vi "Length_10.vi"() -> ()   [LabVIEW 2020]
uses:
  Support/Controls/Cmd_Mouse Popup.ctl
  Support/Controls/Clst_Initialize Input.ctl
  Support/Controls/Clst_Result inspec.ctl
  Support/Controls/Cmd_Var Data IO.ctl
  Variables/Global_Cal Info.vi
panel:
  in  "주파수단위":string(combo)="kHz"
  in  "주파수":string
  in  "입력단위":string(combo)="DC"
  in  "Measured ADJ":string[][](table) caption="조정후"
  out "STD set":string[][](table) caption="○ 기준기 조합 (값)"
  in  "입력전압":dbl=10.0
  in  "정격출력":dbl=10.0
  in  "최소출력":dbl
  in  "출력단위":string(combo)="V"
  out "최소범위":string
  out "Resolution":string[][](table) caption="Spec"
  in  "Spec 변경":bool
  in  "Random":bool
  out "Spec":string[][](table)
  out "제목":string
  out "에러 출력":errorcluster
  out "Condition":string[][](table)
  out "최소눈금":string
  out "단위":string
  out "최대범위":string
  in  "Measured":string[][](table) caption="조정전"
  out "Load?":bool
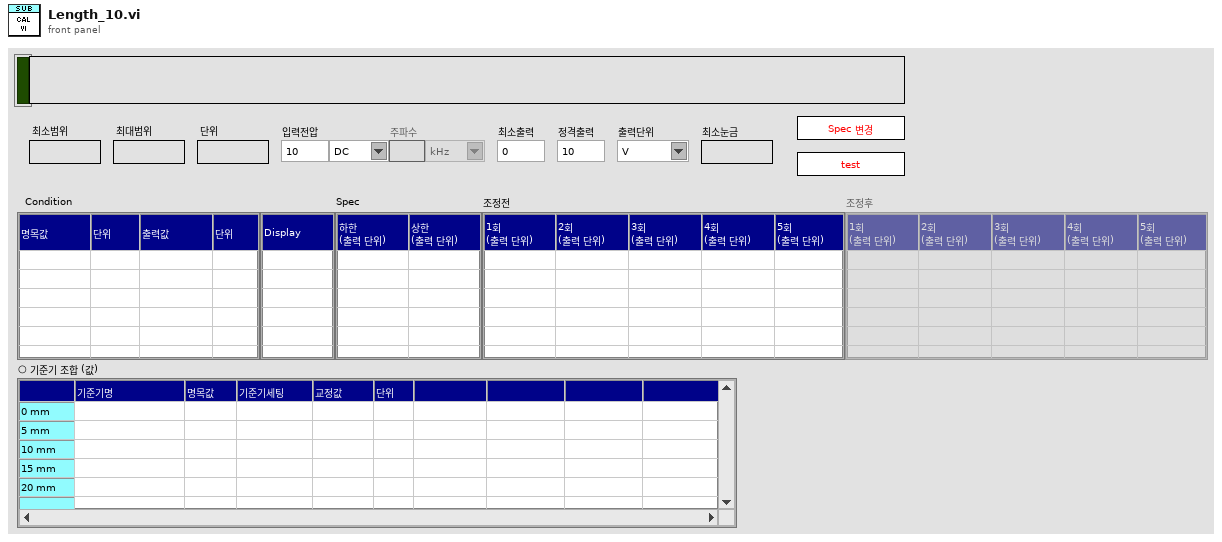
[diagram p1: front panel]
types:
  T1 = typedef "Cmd_Mouse Popup.ctl" = enum16{"활성화", "메뉴선택"}
  T2 = cluster{"Shift":bool, "Ctrl":bool, "Alt":bool, "Cmd":bool, "Opt":bool}
  T3 = typedef "Clst_Initialize Input.ctl" = cluster{"Initialize 1":cluster{"Condition":refnum<vi>[], "Spec":refnum<vi>[], "Measured":refnum<vi>[], "Resolution":refnum<vi>[], "Func_ext":string, "제목":refnum<vi>, "Measured_ADJ":refnum<vi>[]}, "Initialize 2":cluster{"문자열":refnum<vi>[], "콤보박스":refnum<vi>[], "링":refnum<vi>[], "열거형":refnum<vi>[], "테이블":refnum<vi>[], "여러열":refnum<vi>[], "디지털(DBL)":refnum<vi>[], "3D string":refnum<vi>[], "ctrl":refnum<vi>[], "boolean":refnum<vi>[]}}
  T4 = typedef "Clst_Result inspec.ctl" = cluster{"분해능":string, "문자열 1":string, "문자열 2":string, "숫자형 1":i32, "숫자형 2":i32, "숫자형 3":dbl, "문자배열 1D":string[], "문자배열 2D":string[][], "문자배열 3D":string[][][], "문자배열 4D":string[][][][], "불리언 1D":bool[]}
  T5 = typedef "Cmd_Var Data IO.ctl" = enum16{"Condition", "Condition Default", "Condition_Temp", "Resolution", "Resolution Default", "Resolution Old", "Spec", "Spec Default", "Spec Old", "Spec Temp", "Result", "Result2", "Result3", "Result_Temp", "Result_ADJ", "Result_ADJ2", "STD1", "STD2", "STD3", "STD4", "STD5", "STD Temp", "CMC", "CMC Default"}
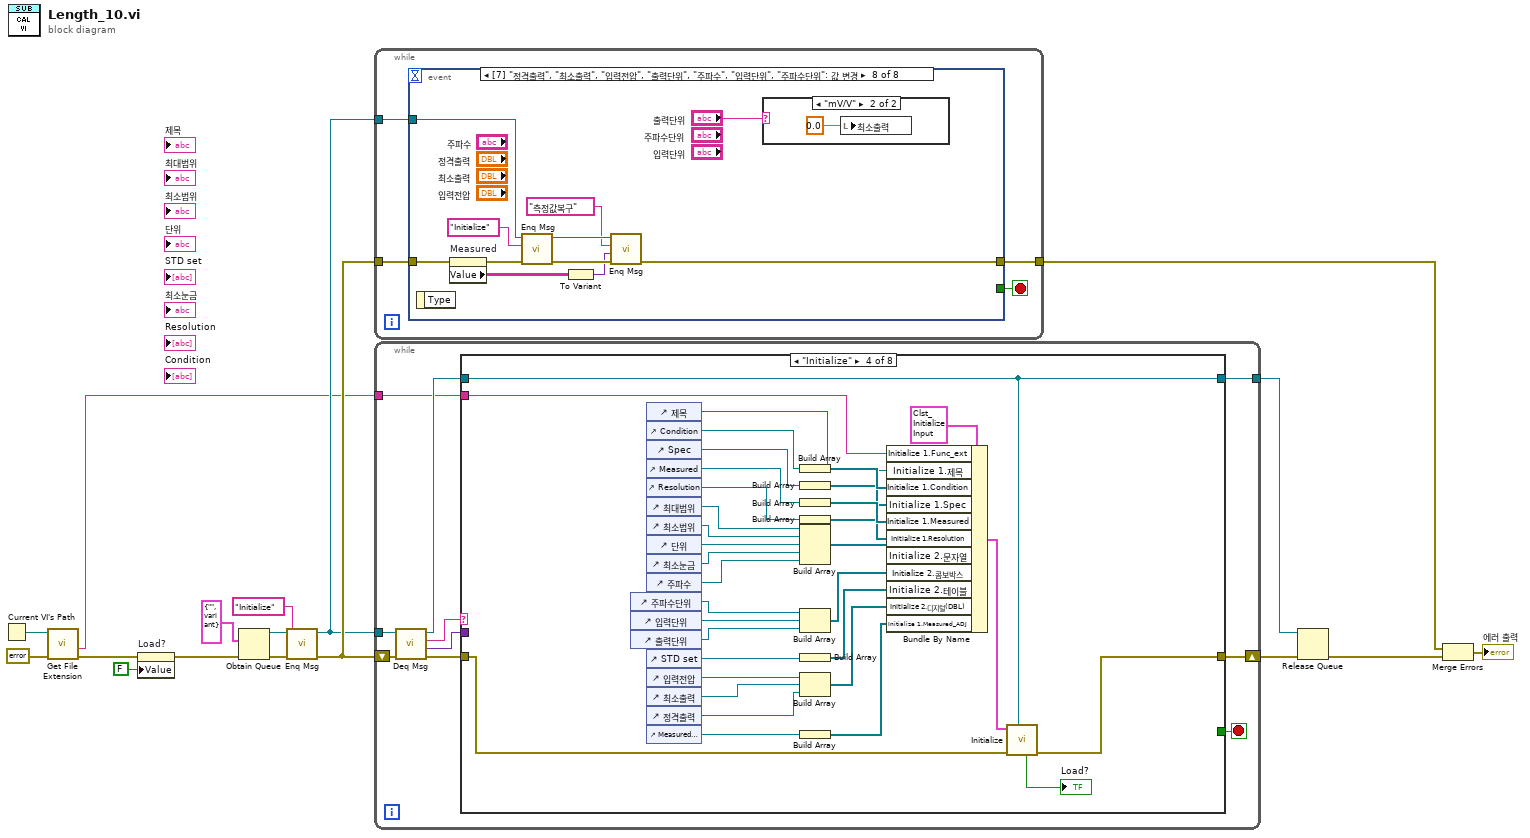
[diagram p0: block diagram]
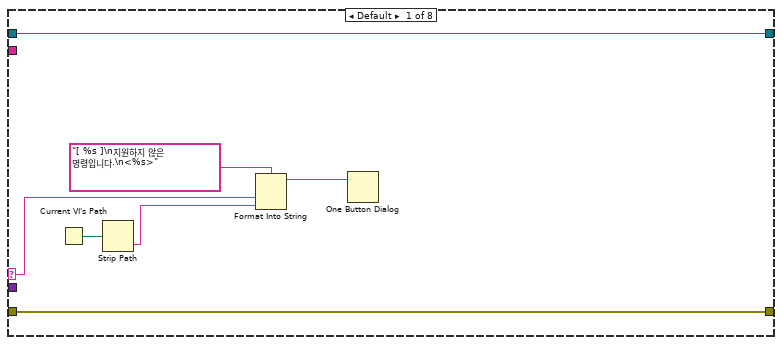
[diagram p2: hidden frame]
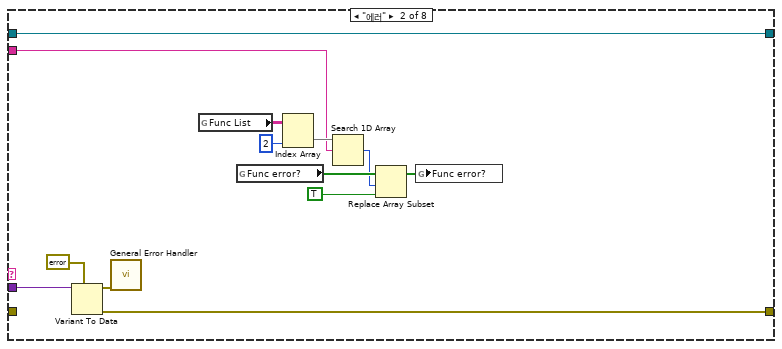
[diagram p3: hidden frame]
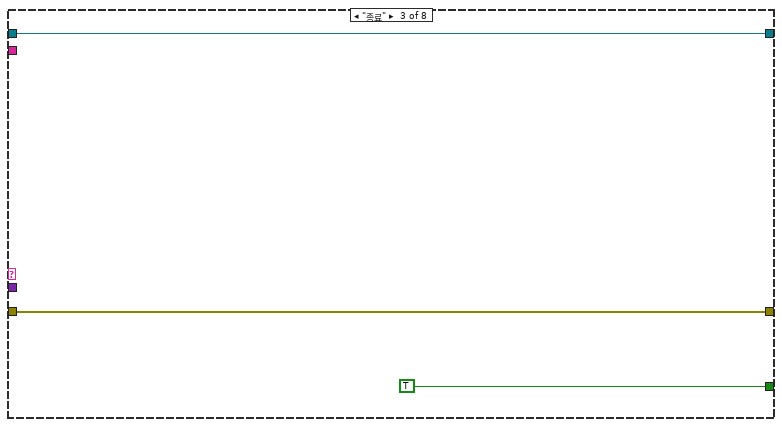
[diagram p4: hidden frame]
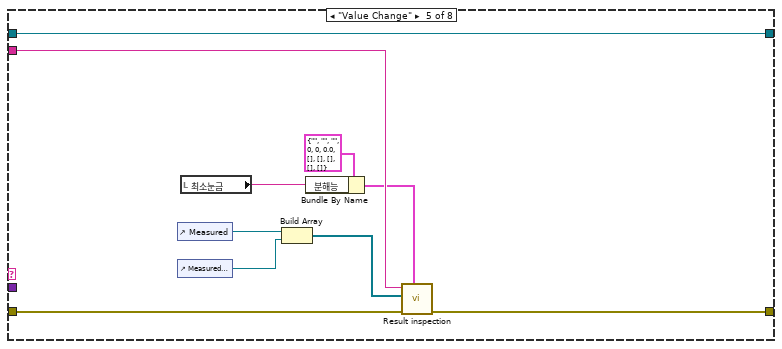
[diagram p5: hidden frame]
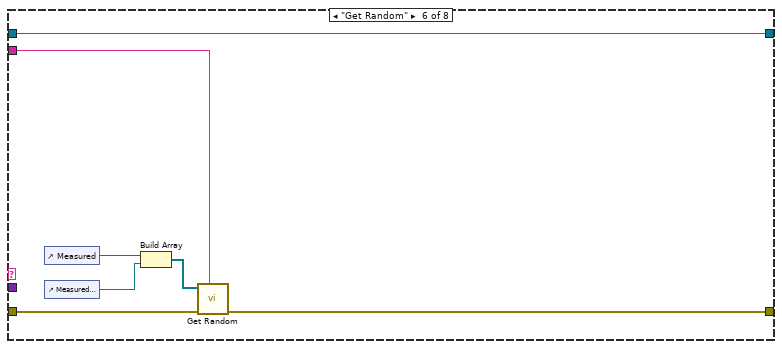
[diagram p6: hidden frame]
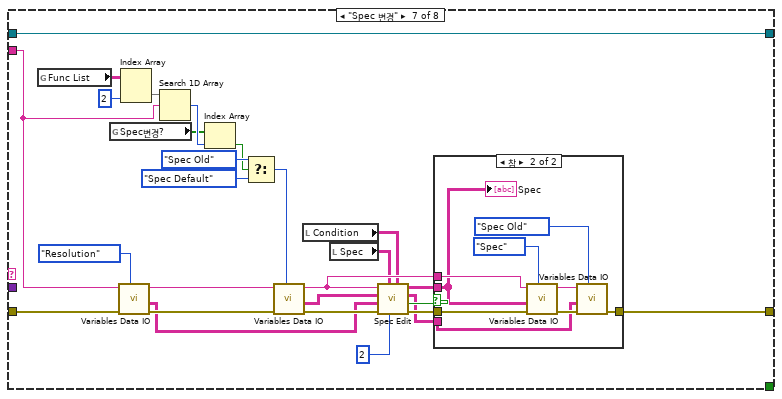
[diagram p7: hidden frame]
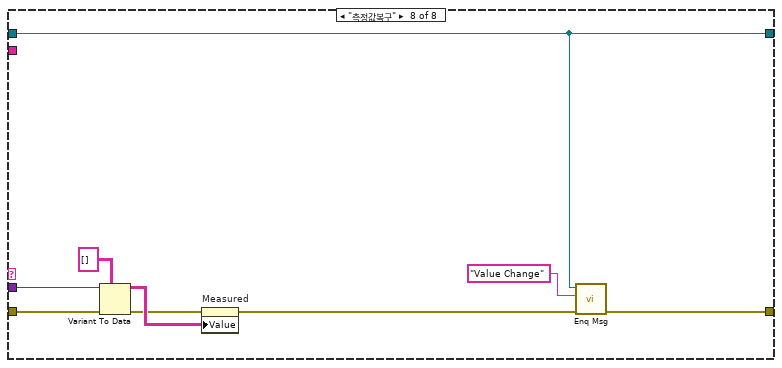
[diagram p9: hidden frame]
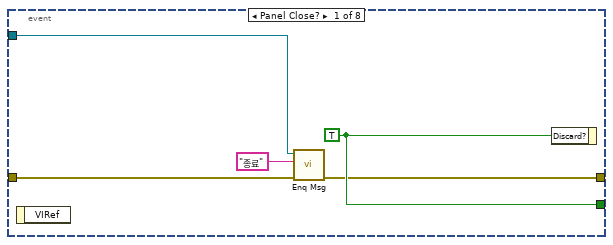
[diagram p10: hidden frame]
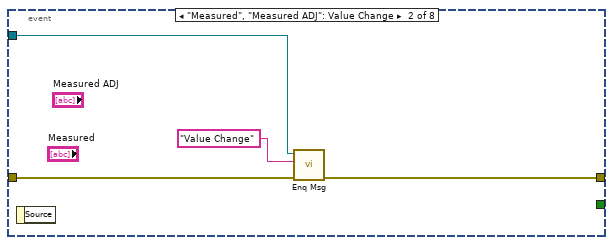
[diagram p11: hidden frame]
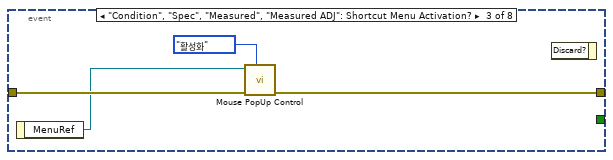
[diagram p12: hidden frame]
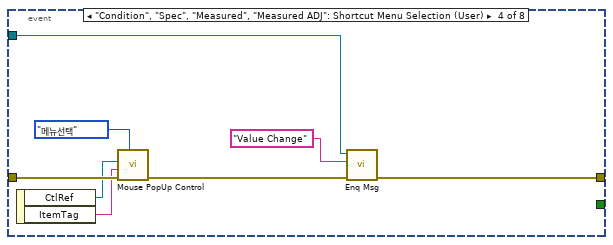
[diagram p13: hidden frame]
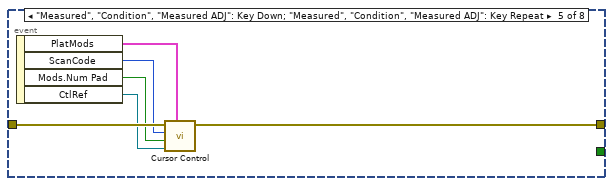
[diagram p14: hidden frame]
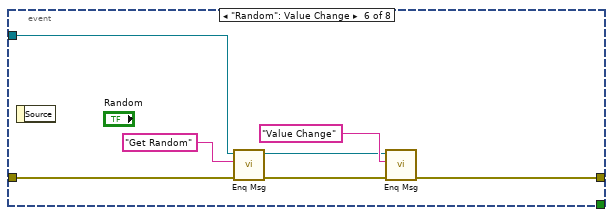
[diagram p15: hidden frame]
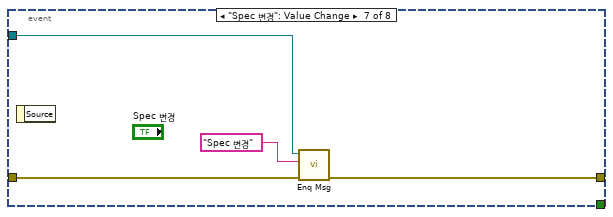
[diagram p16: hidden frame]
diagram:
  n1 = Current VI's Path() -> (path=w7:path)
  n2 = call <vilib>:"Get File Extension.vi"("error in (no error)"=errorcluster {"status"=FALSE, "code"=0, "source"=""} ("에러 상수"), "file"=w7) -> ("error out"=w3:errorcluster, "filename without extension"=w6:string)  [unwired: 5 in, 3 out]
  n3 = property on="Load?" class="Bool (엄격한)"(error in=w3, "Value"=FALSE ("Load?")) -> (error out=w2:errorcluster)  [unwired: 1 in, 1 out]
  n4 = Obtain Queue(element data type=cluster{"메세지":string, "값":variant} {"메세지"="", "값"=variant} ("Message Cluster"), error in (no error)=w2) -> (queue out=w15:refnum<queue>, error out=w5:errorcluster)  [unwired: 3 in, 1 out]
  n5 = call "Enq Msg.vi"("에러 입력(에러 없음)"=w5, "메세지"="Initialize", "큐 입력"=w15) -> ("에러 출력"=w16:errorcluster, "큐 출력"=w13:refnum<queue>)  [unwired: 7 in]
  n6 = while {
    tunnel: w16 -> [w19]
    tunnel: w13 -> [w20]
    tunnel: [w18] -> w10
    stop <- w21 stop-if-true
    n7 = event shown="[7] \"정격출력\", \"최소출력\", \"입력전압\", \"출력단위\", \"주파수\", \"입력단위\", \"주파수단위\": 값 변경" {
      selector: _ -> [_ _ _ _ _ _ _ _]
      dyn-events: _ -> [_ _ _ _ _ _ _ _]
      timeout: _ -> [_ _ _ _ _ _ _ _]
      tunnel: [w26 _ _ _ _ _ _ _] -> w21
      tunnel: w20 -> [w24 w29 _ w37 _ w50 w56 w69]
      tunnel: w19 -> [w25 w30 w33 w41 w48 w51 w58 w67]
      tunnel: [w22 w28 w32 w36 w47 w49 w57 w60] -> w18
      event Panel Close? {
        w26 = TRUE ("버림?")
        n8 = event-data() -> ()  [unwired: 1 in, 1 out]
        n9 = call "Enq Msg.vi"("에러 입력(에러 없음)"=w25, "메세지"="종료", "큐 입력"=w24) -> ("에러 출력"=w22:errorcluster)  [unwired: 7 in, 1 out]
        n10 = event-data("Discard?"=w26) -> ()  [unwired: 1 in, 1 out]
      }
      event "Measured", "Measured ADJ": Value Change {
        n11 = event-data() -> ()  [unwired: 1 in, 1 out]
        n12 = call "Enq Msg.vi"("에러 입력(에러 없음)"=w30, "메세지"="Value Change", "큐 입력"=w29) -> ("에러 출력"=w28:errorcluster)  [unwired: 7 in, 1 out]
      }
      event "Condition", "Spec", "Measured", "Measured ADJ": Shortcut Menu Activation? {
        n13 = event-data() -> ("MenuRef"=w31:refnum<k9>)  [unwired: 1 in]
        n14 = call "Mouse PopUp Control.vi"("type"=Cmd_Mouse_Popup."활성화", "error in"=w33, "메뉴 참조"=w31) -> ("error out"=w32:errorcluster)  [unwired: 8 in]
        n15 = event-data() -> ()  [unwired: 2 in, 1 out]
      }
      event "Condition", "Spec", "Measured", "Measured ADJ": Shortcut Menu Selection (User) {
        n16 = event-data() -> ("CtlRef"=w39:refnum<vi>, "ItemTag"=w40:string)  [unwired: 1 in]
        n17 = call "Mouse PopUp Control.vi"("type"=Cmd_Mouse_Popup."메뉴선택", "error in"=w41, "아이템 태그"=w40, "Tbl 참조 번호"=w39) -> ("error out"=w38:errorcluster)  [unwired: 7 in]
        n18 = call "Enq Msg.vi"("에러 입력(에러 없음)"=w38, "메세지"="Value Change", "큐 입력"=w37) -> ("에러 출력"=w36:errorcluster)  [unwired: 7 in, 1 out]
      }
      event "Measured", "Condition", "Measured ADJ": Key Down; "Measured", "Condition", "Measured ADJ": Key Repeat {
        n19 = event-data() -> ("PlatMods"=w43:T2, "ScanCode"=w46:i16, "Mods.Num Pad"=w45:bool, "CtlRef"=w44:refnum<vi>)  [unwired: 1 in]
        n20 = call "Cursor Control.vi"("플랫폼 조합키"=w43, "참조"=w44, "Num Pad"=w45, "ScanCode"=w46, "error in"=w48) -> ("error out"=w47:errorcluster)  [unwired: 5 in, 1 out]
      }
      event "Random": Value Change {
        n21 = event-data() -> ()  [unwired: 1 in, 1 out]
        n22 = call "Enq Msg.vi"("에러 입력(에러 없음)"=w51, "메세지"="Get Random", "큐 입력"=w50) -> ("에러 출력"=w53:errorcluster, "큐 출력"=w54:refnum<queue>)  [unwired: 7 in]
        n23 = call "Enq Msg.vi"("에러 입력(에러 없음)"=w53, "메세지"="Value Change", "큐 입력"=w54) -> ("에러 출력"=w49:errorcluster)  [unwired: 7 in, 1 out]
      }
      event "Spec 변경": Value Change {
        n24 = event-data() -> ()  [unwired: 1 in, 1 out]
        n25 = call "Enq Msg.vi"("에러 입력(에러 없음)"=w58, "메세지"="Spec 변경", "큐 입력"=w56) -> ("에러 출력"=w57:errorcluster)  [unwired: 7 in, 1 out]
      }
      event "정격출력", "최소출력", "입력전압", "출력단위", "주파수", "입력단위", "주파수단위": Value Change {
        n26 = event-data() -> ()  [unwired: 1 in, 1 out]
        n27 = property on="Measured" class="Tbl (엄격한)"(error in=w67) -> (error out=w66:errorcluster, "Value"=w63:string[][])  [unwired: 1 in, 1 out]
        n28 = call "Enq Msg.vi"("에러 입력(에러 없음)"=w66, "메세지"="Initialize", "큐 입력"=w69) -> ("에러 출력"=w65:errorcluster, "큐 출력"=w68:refnum<queue>)  [unwired: 7 in]
        n29 = To Variant(anything=w63) -> (Variant=w62:variant)
        n30 = call "Enq Msg.vi"("에러 입력(에러 없음)"=w65, "값"=w62, "메세지"="측정값복구", "큐 입력"=w68) -> ("에러 출력"=w60:errorcluster)  [unwired: 6 in, 1 out]
        n31 = case shown="\"mV/V\"" "출력단위" {
          frame Default {
          }
          frame "mV/V" {
            n32 = local write "최소출력"(0.0 ("최소출력")) -> ()
          }
        }
      }
    }
  }
  n33 = while {
    shift-right: [w81] -> w12
    shift-left: w16 -> [w80]
    tunnel: w13 -> [w78]
    tunnel: [w73] -> w11
    tunnel: w6 -> [w72]
    stop <- w74 stop-if-true
    n34 = call "Deq Msg.vi"("에러 입력(에러 없음)"=w80, "큐 입력"=w78) -> ("에러 출력"=w79:errorcluster, "값"=w75:variant, "메세지"=w77:string, "큐 출력"=w76:refnum<queue>)  [unwired: 6 in]
    n35 = case shown="\"Initialize\"" w77 {
      selector: w77 -> [w84 _ _ _ _ _ _ _]
      tunnel: w79 -> [w88 _ w104 w113 w145 w153 w176 w199]
      tunnel: [w88 w98 w104 w112 w147 w150 w180 w194] -> w81
      tunnel: w76 -> [w87 w97 w102 w125 w148 w155 w182 w193]
      tunnel: w75 -> [_ w99 _ _ _ _ _ w198]
      tunnel: [_ _ TRUE ("버림?") _ _ _ _ _] -> w74
      tunnel: [w87 w97 w102 w125 w148 w155 w182 w193] -> w73
      tunnel: w72 -> [_ w89 _ w121 w146 w151 w157 _]
      frame Default {
        n36 = Current VI's Path() -> (path=w83:path)
        n37 = Strip Path(path=w83) -> (name=w82:string)  [unwired: 1 out]
        n38 = Format Into String(format string="[ %s ]\n지원하지 않은 명령입니다.\n<%s>" ("메시지"), w84, w82) -> (resulting string=w85:string)  [unwired: 2 in, 1 out]
        n39 = One Button Dialog(message=w85) -> ()  [unwired: 1 in, 1 out]
      }
      frame "에러" {
        n40 = Variant To Data(type=errorcluster {"status"=FALSE, "code"=0, "source"=""} ("에러 출력"), Variant=w99) -> (data=w101:errorcluster, error out=w98:errorcluster)  [unwired: 1 in]
        n41 = call <vilib>:"General Error Handler.vi"("error in (no error)"=w101) -> ()  [unwired: 10 in, 5 out]
        n42 = global read "Global_Cal Info.vi" "Func List"() -> (w95:string[][])
        n43 = global read "Global_Cal Info.vi" "Func error?"() -> (w92:bool[])
        n44 = Index Array(array=w95, index (col)=2 ("비활성화된 인덱스 (열)")) -> (element=w94:string[])  [unwired: 1 in]
        n45 = Search 1D Array(1D array=w94, element=w89) -> (index of element=w91:i32)  [unwired: 1 in]
        n46 = Replace Array Subset(array=w92, new element=TRUE ("새 원소/부분배열"), index=w91) -> (w90:bool[])
        n47 = global write "Global_Cal Info.vi" "Func error?"(w90) -> ()
      }
      frame "종료" {
      }
      frame "Initialize" {
        n48 = control-ref of="주파수단위"() -> (w106:refnum<vi>)
        n49 = control-ref of="입력단위"() -> (w105:refnum<vi>)
        n50 = control-ref of="출력단위"() -> (w107:refnum<vi>)
        n51 = control-ref of="제목"() -> (w130:refnum<vi>)
        n52 = control-ref of="Condition"() -> (w136:refnum<vi>)
        n53 = control-ref of="Spec"() -> (w127:refnum<vi>)
        n54 = control-ref of="Measured"() -> (w133:refnum<vi>)
        n55 = control-ref of="Resolution"() -> (w124:refnum<vi>)
        n56 = control-ref of="최대범위"() -> (w129:refnum<vi>)
        n57 = control-ref of="최소범위"() -> (w120:refnum<vi>)
        n58 = control-ref of="단위"() -> (w128:refnum<vi>)
        n59 = control-ref of="최소눈금"() -> (w119:refnum<vi>)
        n60 = control-ref of="주파수"() -> (w108:refnum<vi>)
        n61 = control-ref of="STD set"() -> (w114:refnum<vi>)
        n62 = control-ref of="입력전압"() -> (w118:refnum<vi>)
        n63 = control-ref of="최소출력"() -> (w117:refnum<vi>)
        n64 = control-ref of="정격출력"() -> (w116:refnum<vi>)
        n65 = control-ref of="Measured ADJ"() -> (w111:refnum<vi>)
        n66 = Build Array(w136) -> (w135:refnum<vi>[])
        n67 = Build Array(w127) -> (w126:refnum<vi>[])
        n68 = Build Array(w133) -> (w134:refnum<vi>[])
        n69 = Build Array(w124) -> (w123:refnum<vi>[])
        n70 = Build Array(w129, w120, w128, w119, w108) -> (w132:refnum<vi>[])
        n71 = Build Array(w106, w105, w107) -> (w131:refnum<vi>[])
        n72 = Build Array(w114) -> (w122:refnum<vi>[])
        n73 = Build Array(w118, w117, w116) -> (w115:refnum<vi>[])
        n74 = Build Array(w111) -> (w110:refnum<vi>[])
        n75 = Bundle By Name(cluster=T3 {"Initialize 1"={"Condition"=[], "Spec"=[], "Measured"=[], "Resolution"=[], "Func_ext"="", "제목"=refnum, "Measured_ADJ"=[]}, "Initialize 2"={"문자열"=[], "콤보박스"=[], "링"=[], "열거형"=[], "테이블"=[], "여러열"=[], "디지털(DBL)"=[], "3D string"=[], "ctrl"=[], "boolean"=[]}} ("입력 클러스터"), "Initialize 1.Func_ext"=w121, "Initialize 1.제목"=w130, "Initialize 1.Condition"=w135, "Initialize 1.Spec"=w126, "Initialize 1.Measured"=w134, "Initialize 1.Resolution"=w123, "Initialize 2.문자열"=w132, "Initialize 2.콤보박스"=w131, "Initialize 2.테이블"=w122, "Initialize 2.디지털(DBL)"=w115, "Initialize 1.Measured_ADJ"=w110) -> (w137:T3)
        n76 = call "Initialize.vi"("큐 입력"=w125, "error in"=w113, "입력 클러스터"=w137) -> ("error out"=w112:errorcluster, "Load?"=→"Load?":bool)  [unwired: 5 in, 2 out]
      }
      frame "Value Change" {
        n77 = control-ref of="Measured"() -> (w144:refnum<vi>)
        n78 = control-ref of="Measured ADJ"() -> (w139:refnum<vi>)
        n79 = local read "최소눈금"() -> (w141:string)
        n80 = Build Array(w144, w139) -> (w143:refnum<vi>[])
        n81 = Bundle By Name(cluster=T4 {"분해능"="", "문자열 1"="", "문자열 2"="", "숫자형 1"=0, "숫자형 2"=0, "숫자형 3"=0.0, "문자배열 1D"=[], "문자배열 2D"=[], "문자배열 3D"=[], "문자배열 4D"=[], "불리언 1D"=[]} ("입력 클러스터"), "분해능"=w141) -> (w140:T4)
        n82 = call "Result inspection.vi"("입력 클러스터"=w140, "error in"=w145, "Ref. Data (Inspection)"=w143, "Func ext"=w146) -> ("error out"=w147:errorcluster)  [unwired: 4 in, 3 out]
      }
      frame "Get Random" {
        n83 = control-ref of="Measured"() -> (w152:refnum<vi>)
        n84 = control-ref of="Measured ADJ"() -> (w149:refnum<vi>)
        n85 = Build Array(w152, w149) -> (w154:refnum<vi>[])
        n86 = call "Get Random.vi"("Func_Ext"=w151, "에러 입력"=w153, "Meas"=w154) -> ("에러 출력"=w150:errorcluster)  [unwired: 7 in, 1 out]
      }
      frame "Spec 변경" {
        n87 = global read "Global_Cal Info.vi" "Func List"() -> (w162:string[][])
        n88 = global read "Global_Cal Info.vi" "Spec변경?"() -> (w158:bool[])
        n89 = call "Variables Data IO.vi"("Select"=Cmd_Var_Data_IO."Resolution", "error in"=w176, "Func_ext"=w157) -> ("error out"=w175:errorcluster, "Data Out"=w169:string[][], "Func_ext Out"=w174:string)  [unwired: 6 in]
        n90 = Index Array(array=w162, index (col)=2 ("비활성화된 인덱스 (열)")) -> (element=w160:string[])  [unwired: 1 in]
        n91 = Search 1D Array(1D array=w160, element=w157) -> (index of element=w159:i32)  [unwired: 1 in]
        n92 = Index Array(array=w158, index=w159) -> (element=w163:bool)
        n93 = Select(t=Cmd_Var_Data_IO."Spec Old" ("Select"), s=w163, f=Cmd_Var_Data_IO."Spec Default" ("Select")) -> (s? t:f=w156:T5)
        n94 = call "Variables Data IO.vi"("Select"=w156, "error in"=w175, "Func_ext"=w174) -> ("error out"=w177:errorcluster, "Data Out"=w168:string[][], "Func_ext Out"=w170:string)  [unwired: 6 in]
        n95 = local read "Condition"() -> (w166:string[][])
        n96 = local read "Spec"() -> (w167:string[][])
        n97 = call "Spec Edit.vi"("Condition"=w166, "열번호(기준값)"=2 ("기준열(0)"), "Spec Value"=w167, "에러 입력(에러 없음)"=w177, "Resolution"=w169, "Spec Default"=w168, "Func_ext"=w170) -> ("에러 출력"=w181:errorcluster, "변경?"=w178:bool, "Spec Default out"=w172:string[][], "Spec 출력"=w179:string[][])  [unwired: 1 in]
        n98 = case shown="참" w178 {
          tunnel: w181 -> [w183 w191]
          tunnel: [w183 w187] -> w180
          tunnel: w179 -> [_ w189]
          tunnel: w170 -> [_ w190]
          tunnel: w172 -> [_ w185]
          frame False {
          }
          frame True {
            n99 = call "Variables Data IO.vi"("Select"=Cmd_Var_Data_IO."Spec", "error in"=w191, "Data In"=w189, "Func_ext"=w190) -> ("error out"=w188:errorcluster, "Func_ext Out"=w186:string)  [unwired: 5 in, 1 out]
            n100 = call "Variables Data IO.vi"("Select"=Cmd_Var_Data_IO."Spec Old", "error in"=w188, "Data In"=w185, "Func_ext"=w186) -> ("error out"=w187:errorcluster)  [unwired: 5 in, 2 out]
            "Spec" <- w189
          }
        }
      }
      frame "측정값복구" {
        n101 = Variant To Data(error in=w199, type=string[][] [], Variant=w198) -> (data=w197:string[][], error out=w196:errorcluster)
        n102 = property on="Measured" class="Tbl (엄격한)"(error in=w196, "Value"=w197) -> (error out=w195:errorcluster)  [unwired: 1 in, 1 out]
        n103 = call "Enq Msg.vi"("에러 입력(에러 없음)"=w195, "메세지"="Value Change", "큐 입력"=w193) -> ("에러 출력"=w194:errorcluster)  [unwired: 7 in, 1 out]
      }
    }
  }
  n104 = Release Queue(queue=w11, error in (no error)=w12) -> (error out=w4:errorcluster)  [unwired: 1 in, 2 out]
  n105 = Merge Errors(w10, w4) -> (→"에러 출력":errorcluster)
